vi "Vision Processing.vi"(4 "error in (no error)":errorcluster, 6 "Camera Occurance":refnum<k4>, 7 "Image Size":T1=enum."320x240") -> ()   [LabVIEW 2017]
doc: "This VI runs in parallel to other tasks. It gets images from the camera, processes them for color or shape and use that information to affect robot behavior."
uses:
  <vilib>/Rock Robotics/WPI/Camera/WPI_CameraImageSize.ctl
  Robot Global Data.vi
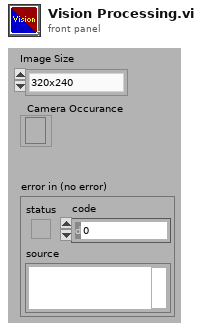
[diagram p1: front panel]
types:
  T1 = typedef "WPI_CameraImageSize.ctl" = enum16{"640x480", "320x240", "160x120", "Custom"}
  T2 = typedef "Image Type" = u32
  T3 = typedef "WPI_CameraDevRef.ctl" = cluster{"Camera Address":string, "CameraStatus":errorcluster}
  T4 = typedef "IMAQ Image.ctl" = refnum<image>
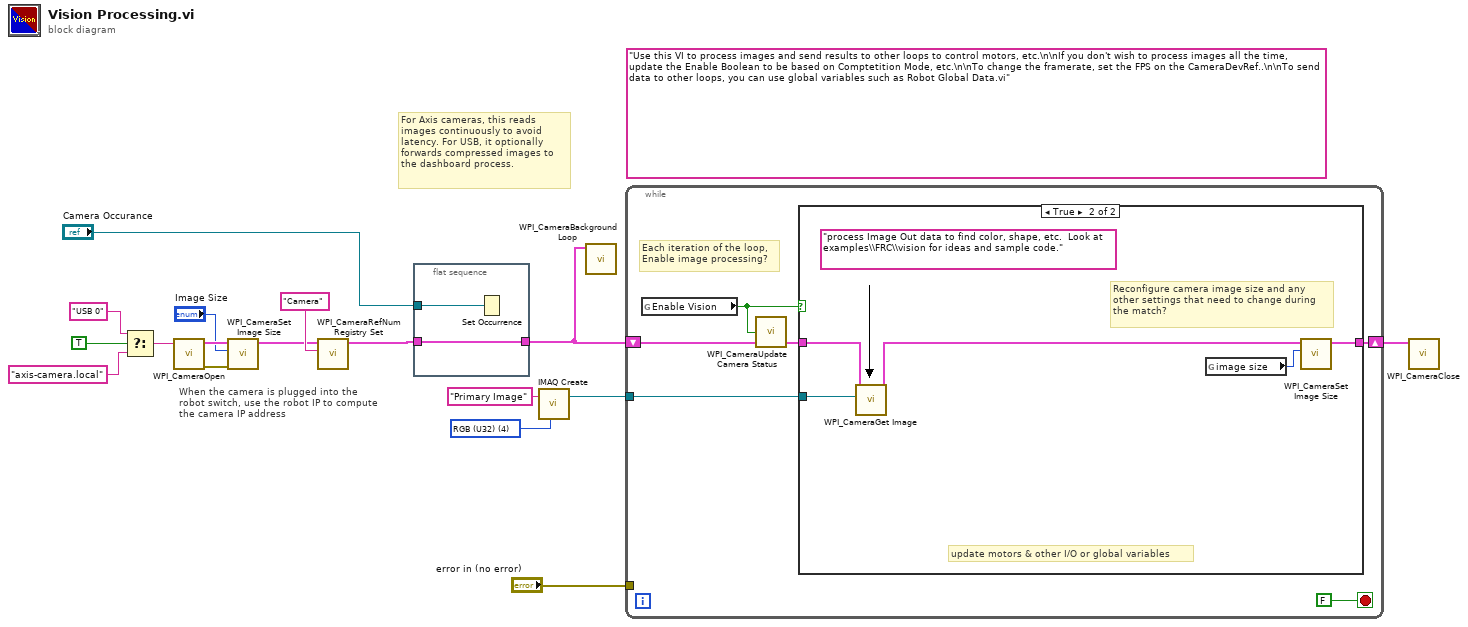
[diagram p0: block diagram]
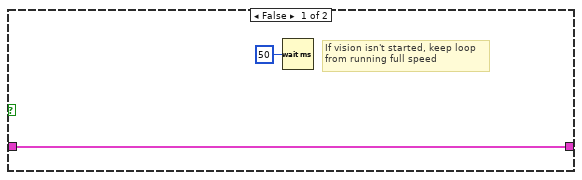
[diagram p2: hidden frame]
diagram:
  (unwired) "Use this VI to process images and send results to other loops to control motors, etc.\n\nIf you don't wish to process images all the time, update the Enable Boolean to be based on Comptetition Mode, etc.\n\nTo change the framerate, set the FPS on the CameraDevRef..\n\nTo send data to other loops, you can use global variables such as Robot Global Data.vi"
  w17 = T2 4 items=["Grayscale (U8)", "Grayscale (I16)", "Grayscale (SGL)", "Complex (CSG)", "RGB (U32)", "HSL (U32)", "RGB (U64)"] ("Image Type")
  # "When the camera is plugged into the\nrobot switch, use the robot IP to compute\nthe camera IP address"
  # "For Axis cameras, this reads\nimages continuously to avoid\nlatency. For USB, it optionally\nforwards compressed images to\nthe dashboard process."
  n1 = Select(t="USB 0" ("format string"), s=TRUE ("dot notation? (F)"), f="axis-camera.local" ("format string")) -> (s? t:f=w6:string)
  n2 = call <vilib>:"WPI_CameraOpen.vi"("Camera Address"=w6) -> ("error out"=w12:errorcluster, "CameraDevRef"=w13:T3)  [unwired: 1 in, 8 out]
  n3 = call <vilib>:"WPI_CameraSet Image Size.vi"("error in (no error)"=w12, "Image Size"="Image Size", "CameraDevRef"=w13) -> ("CameraDevRef Out"=w4:T3)  [unwired: 1 in, 7 out]
  n4 = call <vilib>:"WPI_CameraRefNum Registry Set.vi"("refnum name"="Camera", "CameraDevRef"=w4) -> ("CameraDevRef"=w3:T3)  [unwired: 2 in, 7 out]
  n5 = flat-sequence {
    tunnel: w3 -> [w19]
    tunnel: [w19] -> w2
    tunnel: "Camera Occurance" -> [w18]
    frame #0 {
      n6 = Set Occurrence(w18) -> ()
    }
  }
  n7 = call "IMAQ Create"("Image Name"="Primary Image", "Image Type"=w17) -> ("New Image"=w15:T4)  [unwired: 2 in, 2 out]
  n8 = call <vilib>:"WPI_CameraBackground Loop.vi"("CameraDevRef"=w2) -> ()  [unwired: 11 in]
  n9 = while {
    shift-right: [w24] -> w10
    shift-left: w2 -> [w22]
    tunnel: w15 -> [w23]
    tunnel: "error in (no error)" -> [_]
    stop <- FALSE stop-if-true
    # "Each iteration of the loop,\nEnable image processing?"
    n10 = global read "Robot Global Data.vi" "Enable Vision"() -> (w20:bool)
    n11 = call <vilib>:"WPI_CameraUpdate Camera Status.vi"("CameraDevRef In"=w22, "Enable Vision"=w20) -> ("CameraDevRef Out"=w21:T3)  [unwired: 3 in]
    n12 = case shown="True" w20 {
      tunnel: w23 -> [_ w31]
      tunnel: [w27 w32] -> w24
      tunnel: w21 -> [w27 w29]
      frame False {
        # "If vision isn't started, keep loop\nfrom running full speed"
        n13 = Wait (ms)(milliseconds to wait=u32 50) -> ()  [unwired: 1 out]
      }
      frame True {
        (unwired) "process Image Out data to find color, shape, etc.  Look at examples\\FRC\\vision for ideas and sample code."
        # "update motors & other I/O or global variables"
        # "Reconfigure camera image size and any\nother settings that need to change during\nthe match?"
        n14 = call <vilib>:"WPI_CameraGet Image.vi"("Image"=w31, "CameraDevRef"=w29) -> ("CameraDevRef Out"=w28:T3)  [unwired: 1 in, 8 out]
        n15 = global read "Robot Global Data.vi" "image size"() -> (w30:T1)
        n16 = call <vilib>:"WPI_CameraSet Image Size.vi"("Image Size"=w30, "CameraDevRef"=w28) -> ("CameraDevRef Out"=w32:T3)  [unwired: 2 in, 7 out]
      }
    }
  }
  n17 = call <vilib>:"WPI_CameraClose.vi"("CameraDevRef"=w10) -> ()  [unwired: 1 in, 10 out]
